vi "Send Engine Pointer.vi"(8 "error in (no error)":errorcluster, 10 "Engine Pointer":refnum<class "Memory.Pointer.lvclass">, 11 "Transceiver Interface in":refnum<class "Transceiver Interface.lvclass">) -> (0 "error out":errorcluster, 3 "Transceiver Interface out":refnum<class "Transceiver Interface.lvclass">)   [LabVIEW 2017, in "Data Sharing Framework Engine.lvlib" / "Transceiver Thread.lvclass"]
uses:
  Transceiver Thread.lvclass
  Interfaces/Transceiver Interface/Transceiver Interface.lvclass
  <vilib>/National Instruments/Memory Manager/Classes/Pointer/Memory.Pointer.lvclass
  Interfaces/Transceiver Interface/Command Data.ctl
  Interfaces/Transceiver Interface/Command.ctl
  Interfaces/Transceiver Interface/Command Parameters.ctl
  <vilib>/National Instruments/Memory Manager/Classes/Pointer/Memory.Pointer.lvclass/Memory.Pointer.ctl
  Interfaces/Transceiver Interface/Response.ctl
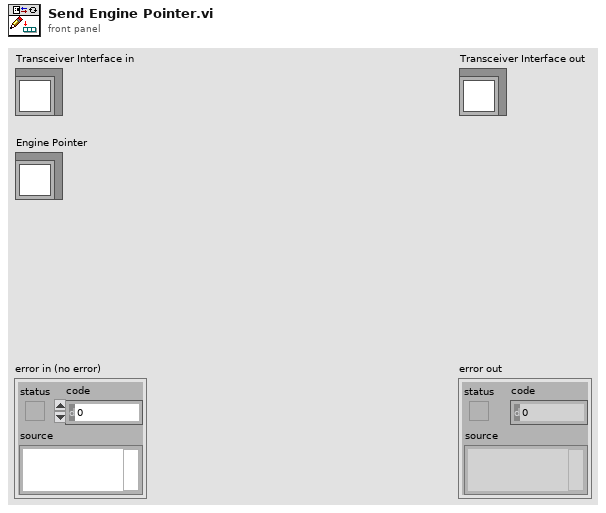
[diagram p1: front panel]
types:
  T1 = typedef "Data Sharing Framework Engine.lvlib/Transceiver Interface.lvclass/Command Data.ctl" = cluster{"Command":T2, "Command Parameters":T3}
  T2 = typedef "Data Sharing Framework Engine.lvlib/Transceiver Interface.lvclass/Command.ctl" = enum8{"Set Base Pointer", "Receive", "Transmit", "Shutdown"}
  T3 = typedef "Data Sharing Framework Engine.lvlib/Transceiver Interface.lvclass/Command Parameters.ctl" = cluster{"arg1":u64, "arg2":u64}
  T4 = typedef "Data Sharing Framework Engine.lvlib/Transceiver Interface.lvclass/Response.ctl" = enum8{"General Ack", "Shutting Down"}
  T5 = typedef "Data Sharing Framework Engine.lvlib/Transceiver Interface.lvclass/Response Data.ctl" = cluster{"Response":T4, "Response Parameters":T6}
  T6 = typedef "Data Sharing Framework Engine.lvlib/Transceiver Interface.lvclass/Response Parameters.ctl" = cluster{"arg1":u64, "arg2":u64}
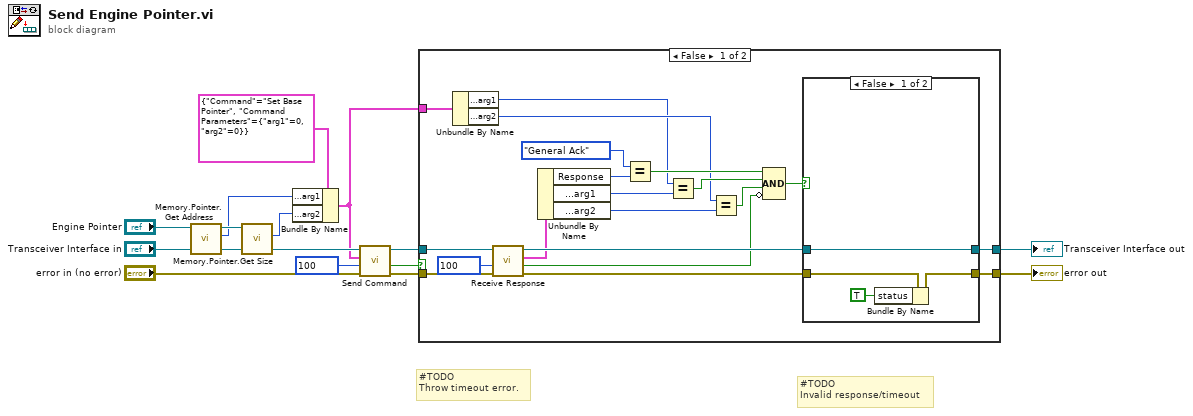
[diagram p0: block diagram]
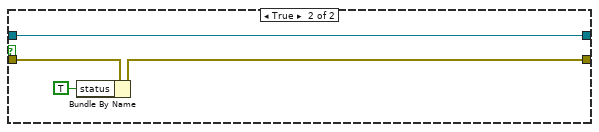
[diagram p3: hidden frame]
diagram:
  # "#TODO\nInvalid response/timeout"
  # "#TODO\nThrow timeout error."
  n1 = call <vilib>:"Memory.Pointer.Get Address.vi"("Pointer in"="Engine Pointer") -> ("address"=w1:u64, "Pointer out"=w3:refnum<class "Memory.Pointer.lvclass">)  [unwired: 9 in]
  n2 = call <vilib>:"Memory.Pointer.Get Size.vi"("Pointer in"=w3) -> ("size"=w2:u64)  [unwired: 9 in, 1 out]
  n3 = Bundle By Name(cluster=T1 {"Command"=enum."Set Base Pointer", "Command Parameters"={"arg1"=0, "arg2"=0}} ("command"), "Command Parameters.arg1"=w1, "Command Parameters.arg2"=w2) -> (w5:T1)
  n4 = call "Send Command.vi"("error in (no error)"="error in (no error)", "timeout in ms (0)"=100, "command"=w5, "Transceiver Interface in"="Transceiver Interface in") -> ("error out"=w12:errorcluster, "timed out?"=w13:bool, "Transceiver Interface out"=w11:refnum<class "Transceiver Interface.lvclass">)  [unwired: 5 in]
  n5 = case shown="False" w13 {
    tunnel: w12 -> [w33 w44]
    tunnel: w11 -> [w34 w41]
    tunnel: [w26 w42] -> w8
    tunnel: [w24 w41] -> w7
    tunnel: w5 -> [w21 _]
    frame False {
      n6 = Unbundle By Name(w21) -> ("Command Parameters.arg1"=w15:u64, "Command Parameters.arg2"=w16:u64)
      n7 = call "Receive Response.vi"("error in (no error)"=w33, "timeout in ms (0)"=100, "Transceiver Thread in"=w34) -> ("error out"=w27:errorcluster, "timed out?"=w22:bool, "response"=w23:T5, "Transceiver Thread out"=w25:refnum<class "Transceiver Interface.lvclass">)  [unwired: 5 in]
      n8 = Unbundle By Name(w23) -> ("Response"=w31:T4, "Response Parameters.arg1"=w20:u64, "Response Parameters.arg2"=w19:u64)
      n9 = Equal?(x=Response."General Ack", y=w31) -> (x = y?=w29:bool)
      n10 = Equal?(x=w15, y=w20) -> (x = y?=w18:bool)
      n11 = Equal?(x=w16, y=w19) -> (x = y?=w17:bool)
      n12 = Compound Arithmetic op=AND(w29, w18, w17, invert w22) -> (w28:bool)
      n13 = case shown="False" w28 {
        tunnel: w27 -> [w38 w40]
        tunnel: [w36 w40] -> w26
        tunnel: w25 -> [w35 w39]
        tunnel: [w35 w39] -> w24
        frame False {
          n14 = Bundle By Name(cluster=w38, "status"=TRUE) -> (w36:errorcluster)
        }
        frame True {
        }
      }
    }
    frame True {
      n15 = Bundle By Name(cluster=w44, "status"=TRUE) -> (w42:errorcluster)
    }
  }
  "error out" <- w8
  "Transceiver Interface out" <- w7
